vi "h3_renkbelirle.vi"(0 "?":string) -> (1 "Frame Color":u32(colorbox), 2 "Voltage Digit Color":u32(colorbox), 3 "Outflow Tube":u32(colorbox), 4 "Current Digit Color":u32(colorbox))   [LabVIEW 2023]
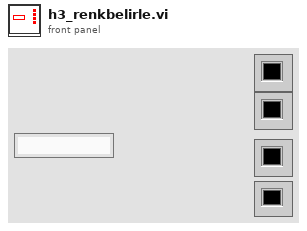
[diagram p1: front panel]
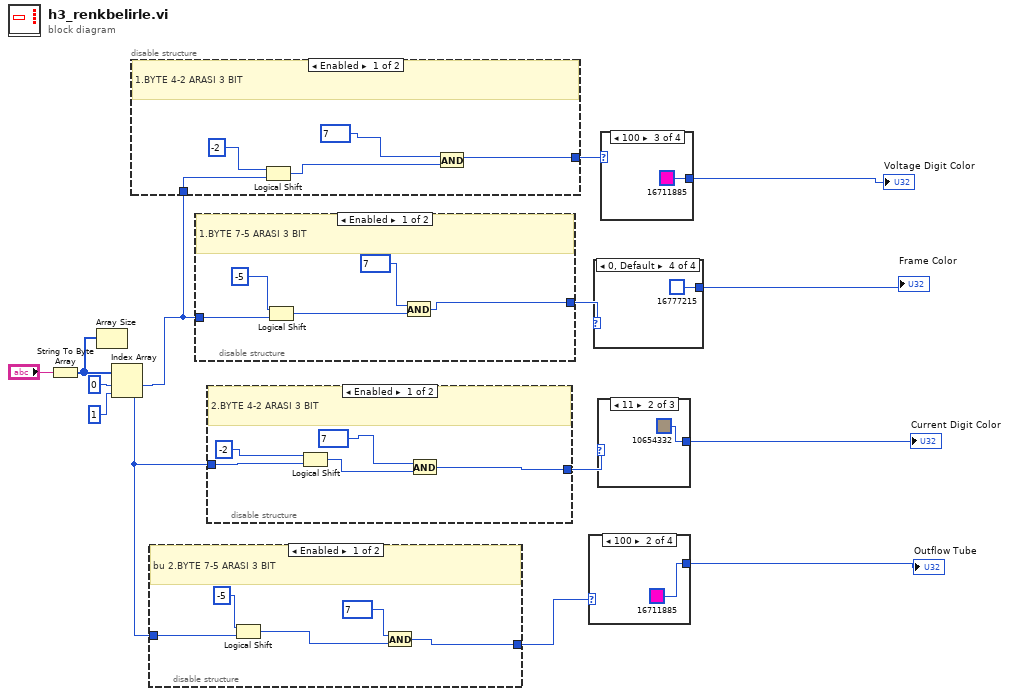
[diagram p0: block diagram]
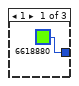
[diagram p6: hidden frame]
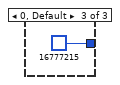
[diagram p7: hidden frame]
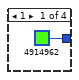
[diagram p8: hidden frame]
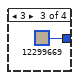
[diagram p9: hidden frame]
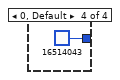
[diagram p10: hidden frame]
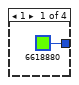
[diagram p11: hidden frame]
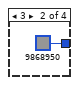
[diagram p12: hidden frame]
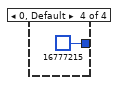
[diagram p13: hidden frame]
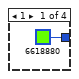
[diagram p14: hidden frame]
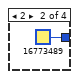
[diagram p15: hidden frame]
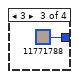
[diagram p16: hidden frame]
diagram:
  n1 = String To Byte Array(string="?") -> (unsigned byte array=w3:u8[])
  n2 = Array Size(array=w3) -> ()  [unwired: 1 out]
  n3 = Index Array(array=w3, index #1=0 ("index"), index #2=1 ("index")) -> (element #1=w1:u8, element #2=w4:u8)
  n4 = disable-structure shown="Enabled" {
    disable-tunnel: [w17 _] -> w9
    disable-tunnel: w1 -> [w16 _]
    frame Enabled {
      # "1.BYTE 4-2 ARASI 3 BIT"
      n5 = Logical Shift(y=i16 -2, x=w16) -> (x << y=w18:u8)
      n6 = And(x=u8 7, y=w18) -> (x .and. y?=w17:u8)
    }
    frame Disabled {
    }
  }
  n7 = disable-structure shown="Enabled" {
    disable-tunnel: [w22 _] -> w7
    disable-tunnel: w4 -> [w20 _]
    frame Enabled {
      # "bu 2.BYTE 7-5 ARASI 3 BIT"
      n8 = Logical Shift(y=i16 -5, x=w20) -> (x << y=w21:u8)
      n9 = And(x=u8 7, y=w21) -> (x .and. y?=w22:u8)
    }
    frame Disabled {
    }
  }
  n10 = disable-structure shown="Enabled" {
    disable-tunnel: [w27 _] -> w10
    disable-tunnel: w1 -> [w25 _]
    frame Enabled {
      # "1.BYTE 7-5 ARASI 3 BIT"
      n11 = Logical Shift(y=i16 -5, x=w25) -> (x << y=w26:u8)
      n12 = And(x=u8 7, y=w26) -> (x .and. y?=w27:u8)
    }
    frame Disabled {
    }
  }
  n13 = disable-structure shown="Enabled" {
    disable-tunnel: [w32 _] -> w5
    disable-tunnel: w4 -> [w31 _]
    frame Enabled {
      # "2.BYTE 4-2 ARASI 3 BIT"
      n14 = Logical Shift(y=i16 -2, x=w31) -> (x << y=w33:u8)
      n15 = And(x=u8 7, y=w33) -> (x .and. y?=w32:u8)
    }
    frame Disabled {
    }
  }
  n16 = case shown="100" w7 {
    tunnel: [u32 4914962 u32 16711885 u32 12299669 u32 16514043] -> w8
    frame 1 {
    }
    frame 4 {
    }
    frame 3 {
    }
    frame 0, Default {
    }
  }
  "Outflow Tube" <- w8
  n17 = case shown="0, Default" w10 {
    tunnel: [u32 6618880 u32 16773489 u32 11771788 u32 16777215] -> w11
    frame 1 {
    }
    frame 2 {
    }
    frame 3 {
    }
    frame 0, Default {
    }
  }
  "Frame Color" <- w11
  n18 = case shown="11" w5 {
    tunnel: [u32 6618880 u32 10654332 u32 16777215] -> w6
    frame 1 {
    }
    frame 3 {
    }
    frame 0, Default {
    }
  }
  "Current Digit Color" <- w6
  n19 = case shown="100" w9 {
    tunnel: [u32 6618880 u32 9868950 u32 16711885 u32 16777215] -> w2
    frame 1 {
    }
    frame 3 {
    }
    frame 4 {
    }
    frame 0, Default {
    }
  }
  "Voltage Digit Color" <- w2
